vi "Make string.vi"(8 "error in (no error)":errorcluster, 11 "Construct String Header in":refnum<class "Construct String Header.lvclass">) -> (0 "error out":errorcluster, 2 "String Header":string, 3 "Construct String Header out":refnum<class "Construct String Header.lvclass">)   [LabVIEW 2018, in "Construct String Header.lvclass"]
doc: "Este VI realiza a leitura das informações do header da imagem, retornando uma string do header."
uses:
  Construct String Header.lvclass
  Construct String Header.lvclass/Construct String Header.ctl
panel:
  out "Header Contents":T1
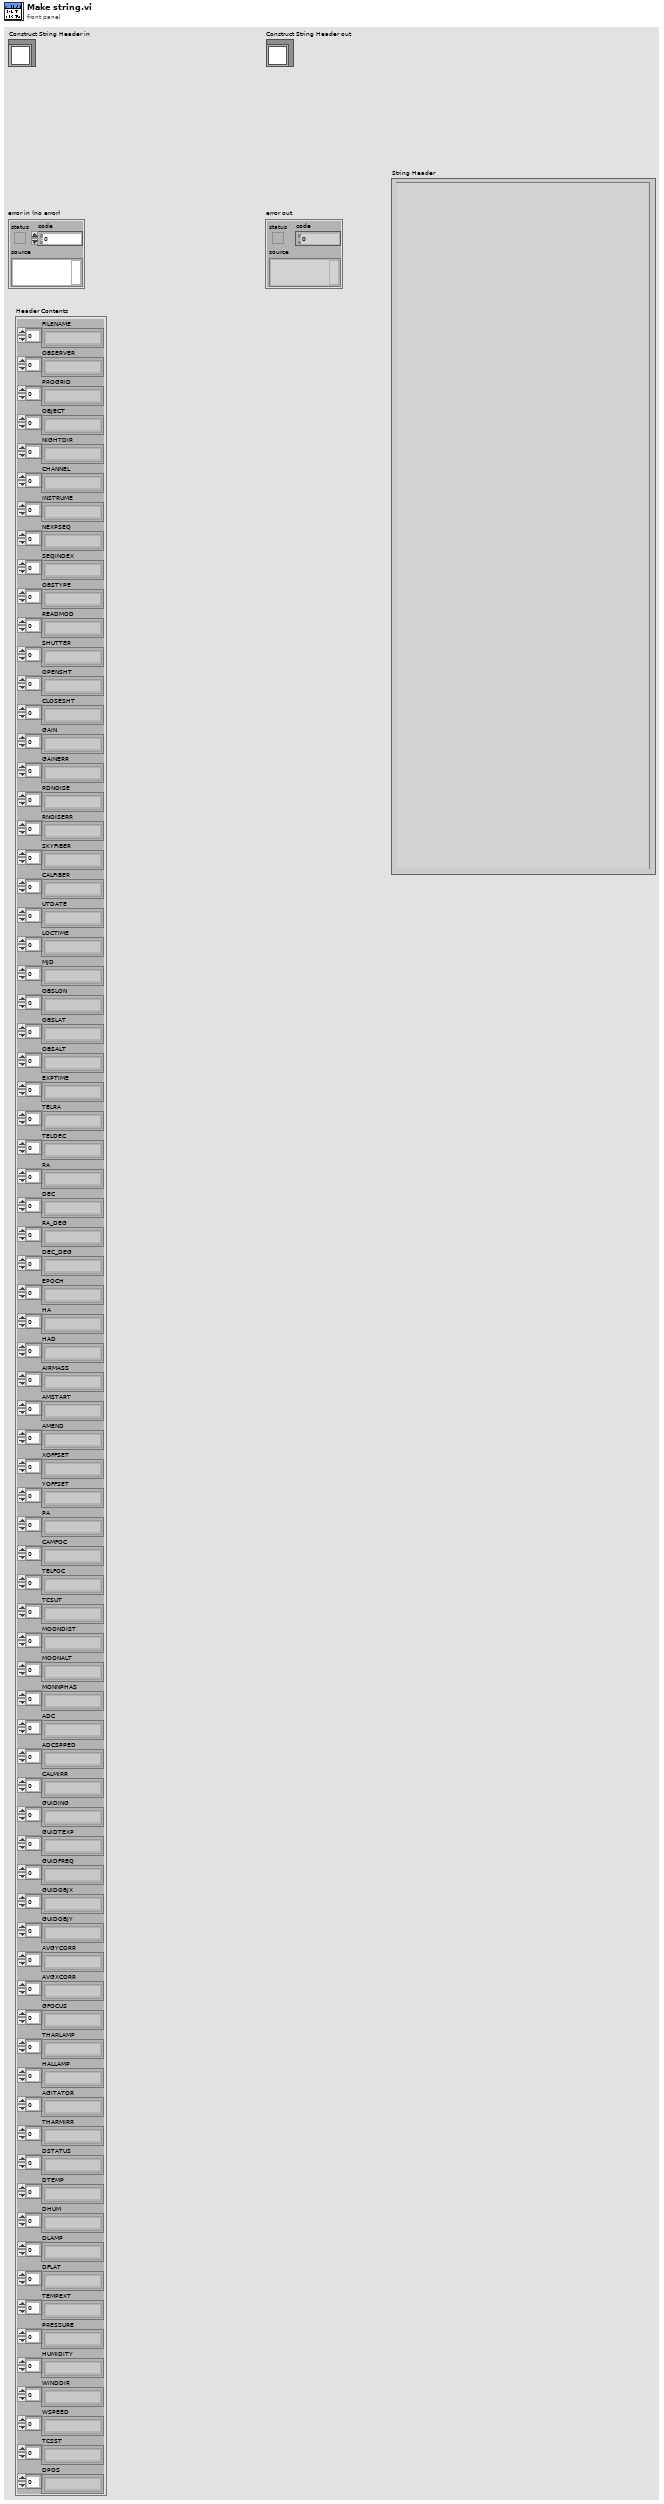
[diagram p1: front panel]
types:
  T1 = cluster{"FILENAME":string[], "OBSERVER":string[], "PROGRID":string[], "OBJECT":string[], "NIGHTDIR":string[], "CHANNEL":string[], "INSTRUME":string[], "NEXPSEQ":string[], "SEQINDEX":string[], "OBSTYPE":string[], "READMOD":string[], "SHUTTER":string[], "OPENSHT":string[], "CLOSESHT":string[], "GAIN":string[], "GAINERR ":string[], "RDNOISE":string[], "RNOISERR":string[], "SKYFIBER":string[], "CALFIBER":string[], "UTDATE":string[], "LOCTIME":string[], "MJD":string[], "OBSLON":string[], "OBSLAT":string[], "OBSALT":string[], "EXPTIME":string[], "TELRA":string[], "TELDEC":string[], "RA":string[], "DEC":string[], "RA_DEG":string[], "DEC_DEG":string[], "EPOCH":string[], "HA":string[], "HAD":string[], "AIRMASS":string[], "AMSTART":string[], "AMEND":string[], "XOFFSET":string[], "YOFFSET":string[], "PA":string[], "CAMFOC":string[], "TELFOC":string[], "TCSUT":string[], "MOONDIST":string[], "MOONALT":string[], "MONNPHAS":string[], "ADC":string[], "ADCSPPED":string[], "CALMIRR":string[], "GUIDING":string[], "GUIDTEXP":string[], "GUIDFREQ":string[], "GUIDOBJX":string[], "GUIDOBJY":string[], "AVGYCORR":string[], "AVGXCORR":string[], "GFOCUS":string[], "THARLAMP":string[], "HALLAMP":string[], "AGITATOR":string[], "THARMIRR":string[], "DSTATUS":string[], "DTEMP":string[], "DHUM":string[], "DLAMP":string[], "DFLAT":string[], "TEMPEXT":string[], "PRESSURE":string[], "HUMIDITY":string[], "WINDDIR":string[], "WSPEED":string[], "TCSST":string[], "DPOS":string[]}
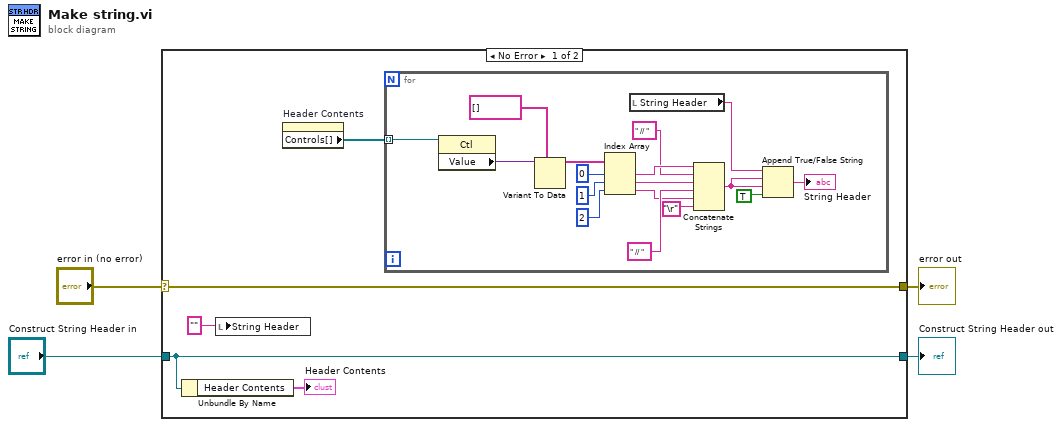
[diagram p0: block diagram]
diagram:
  n1 = case shown="No Error" "error in (no error)" {
    selector: "error in (no error)" -> [w9 w28]
    tunnel: [w9 w28] -> w3
    tunnel: [w8 w27] -> w1
    tunnel: "Construct String Header in" -> [w8 w27]
    frame No Error {
      n2 = Unbundle By Name(w8) -> ("Header Contents"=→"Header Contents":T1)
      n3 = local write "String Header"("") -> ()
      n4 = property on="Header Contents" class="Clust (strict)"() -> ("Controls[]"=w6:refnum<vi>[])  [unwired: 2 in, 2 out]
      n5 = for {
        tunnel: w6 -> [w26] mode=indexing
        n6 = property class="Ctl"(reference=w26) -> ("Value"=w25:variant)  [unwired: 1 in, 2 out]
        n7 = Variant To Data(type=string[] [], Variant=w25) -> (data=w23:string[])  [unwired: 1 in, 1 out]
        n8 = Index Array(array=w23, index #1=0, index #2=1, index #3=2) -> (element #1=w15:string, element #2=w13:string, element #3=w11:string)
        n9 = local read "String Header"() -> (w18:string)
        n10 = Concatenate Strings(w15, " // ", w13, " // ", w11, "\r") -> (w17:string)
        n11 = Append True/False String(1:TRUE ("selector"), 2:w17, 3:w17, 4:w18) -> (0:→"String Header":string)
      }
    }
    frame Error {
    }
  }
  "error out" <- w3
  "Construct String Header out" <- w1
